vi "GetLVQualifiedName.vi"(8 "error in (no error)":errorcluster, 11 "LV File Path":path) -> (0 "error out":errorcluster, 2 "Non LabVIEW File?":bool, 3 "VI Name / CTL Name / LVCLASS Name":string)   [LabVIEW 2019, in "Hawkeye.lvlib"]
uses:
  Hawkeye.lvlib
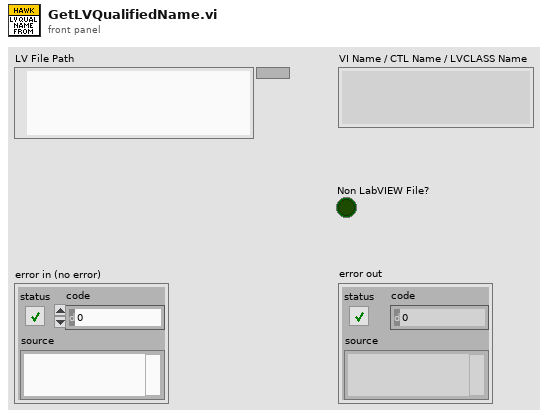
[diagram p1: front panel]
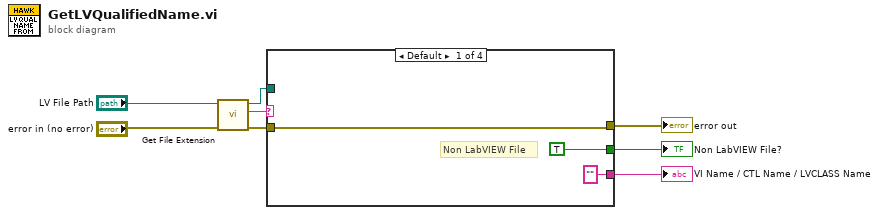
[diagram p0: block diagram]
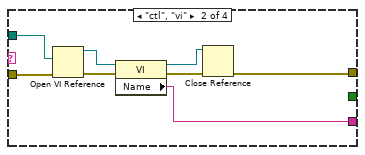
[diagram p2: hidden frame]
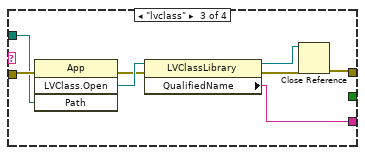
[diagram p3: hidden frame]
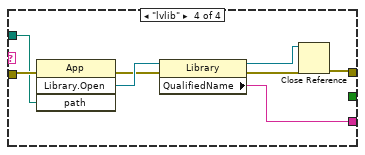
[diagram p4: hidden frame]
diagram:
  n1 = call <vilib>:"Get File Extension.vi"("error in (no error)"="error in (no error)", "file"="LV File Path") -> ("error out"=w8:errorcluster, "lowercase file extension"=w6:string, "dup file"=w7:path)  [unwired: 5 in, 2 out]
  n2 = case shown="Default" w6 {
    tunnel: w7 -> [_ w18 w25 w33]
    tunnel: w8 -> [w11 w19 w26 w34]
    tunnel: [w11 w12 w21 w29] -> w4
    tunnel: ["" ("QualifiedName") w15 w23 w31] -> w1
    tunnel: [TRUE _ _ _] -> w2
    frame Default {
      # "Non LabVIEW File"
    }
    frame "ctl", "vi" {
      n3 = Open VI Reference(vi path=w18, error in (no error)=w19) -> (vi reference=w16:refnum<vi>, error out=w17:errorcluster)  [unwired: 4 in]
      n4 = property on="Property Node" class="VI"(reference=w16, error in=w17) -> (reference out=w13:refnum<vi>, error out=w14:errorcluster, "Name"=w15:string)
      n5 = Close Reference(reference=w13, error in (no error)=w14) -> (error out=w12:errorcluster)
    }
    frame "lvclass" {
      n6 = invoke on="Invoke Node" class="App" method="LVClass.Open"(error in=w26, "Path"=w25) -> (error out=w24:errorcluster, "LVClass.Open"=w27:refnum<vi>)  [unwired: 2 in, 2 out]
      n7 = property on="Property Node" class="LVClassLibrary"(reference=w27, error in=w24) -> (reference out=w20:refnum<vi>, error out=w22:errorcluster, "QualifiedName"=w23:string)
      n8 = Close Reference(reference=w20, error in (no error)=w22) -> (error out=w21:errorcluster)
    }
    frame "lvlib" {
      n9 = invoke on="Invoke Node" class="App" method="Library.Open"(error in=w34, "path"=w33) -> (error out=w32:errorcluster, "Open Library"=w35:refnum<vi>)  [unwired: 2 in, 2 out]
      n10 = property on="Property Node" class="Library"(reference=w35, error in=w32) -> (reference out=w28:refnum<vi>, error out=w30:errorcluster, "QualifiedName"=w31:string)
      n11 = Close Reference(reference=w28, error in (no error)=w30) -> (error out=w29:errorcluster)
    }
  }
  "VI Name / CTL Name / LVCLASS Name" <- w1
  "error out" <- w4
  "Non LabVIEW File?" <- w2
